vi "Stream to TDMS Files.vi"() -> ()   [LabVIEW 2023]
doc: "The Stream to TDMS File example shows how to save images to a TDMS file when using a grab acquisition. The TDMS API has been optimized to take advantage of asynchronous writes, parallel background workers, disk reservation, and disable buffering to improve write perfromance. Read the comments on the block diagram of this VI to learn more about these optimization options."
uses:
  SubVIs/Grab Manager Mode.ctl
  SubVIs/TDMS Write Settings.ctl
  <vilib>/vision/Image Controls.llb/IMAQ Image.ctl
  <vilib>/vision/driver/IMAQdx.llb/IMAQdx Buffer Number Mode.ctl
  <vilib>/Utility/High Resolution Relative Seconds.vi
  SubVIs/TDMS File Initialization (Write).vi
  <vilib>/vision/EDVR.llb/IMAQ ImageToEDVR.vi
  <vilib>/vision/EDVR.llb/IMAQ ImageToEDVR 1D U8.vi
  <vilib>/vision/EDVR.llb/IMAQ ImageToEDVR 1D I16.vi
  <vilib>/vision/EDVR.llb/IMAQ ImageToEDVR 1D U32.vi
  <vilib>/vision/EDVR.llb/IMAQ ImageToEDVR 1D U16.vi
  <vilib>/vision/driver/NI_Vision_Acquisition_Software.lvlib
  <resource>/objmgr/imaqdx.rc
panel:
  out "Optimizations":T1
  in  "Skip Count":u32
  out "Images Saved Per Second":dbl
  out "Images Acquired Per Second":dbl
  in  "Images per TDMS":i64=10000
  out "Write Speed":dbl(graph) caption="Image File Write Speed"
  out "Destination Folder":path
  out "Images Behind":u32
  in  "Number of Images":i32=30
  in  "Camera Name":refnum<k21> caption="IMAQdx Session"
  in  "Stop":bool
  # "Overview: Demonstrates how to stream images to TDMS files when using a grab acquisition.\nRequirements: Vision Acquisition Software\nInstructions:\n1. Select the Camera Name\n2. Run the VI\n3. Increase the Skip Count if Images Behind is greater than 0."
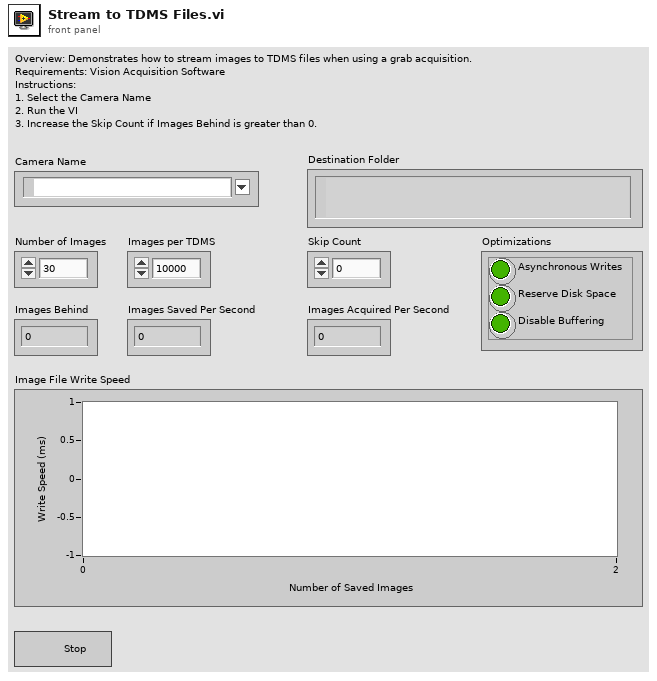
[diagram p1: front panel]
types:
  T1 = cluster{"Asynchronous Writes":bool, "Reserve Disk Space":bool, "Disable Buffering":bool}
  T2 = typedef "TDMS Write Settings.ctl" = cluster{"Asynchronous":bool, "Disable Buffering if Supported":bool, "Reserved Images":i64, "Fail if Reservation Fails":bool}
  T3 = typedef "Grab Manager Mode.ctl" = enum16{"Create Processing Images", "Lock", "Add Acquired Image", "Get Acquired Image", "Unlock", "Dispose Processing Images"}
  T4 = cluster{"Number of Processing Images":u32, "Image Border Size":u32}
  T5 = typedef "IMAQdx.ctl" = refnum<k21>
  T6 = typedef "IMAQ Image.ctl" = refnum<image>
  T7 = typedef "Image Type" = u32
  T8 = cluster{"Image Type":T7, "Async File Format":bool}
  T9 = cluster{"Asynchronous Write":bool, "Reserve Disk Space":bool, "Disable Buffering":bool}
  T10 = typedef "NI_Vision_Acquisition_Software.lvlib/IMAQdx Buffer Number Mode.ctl" = enum32{"Next", "Last", "Buffer Number", "Every", "Last New"}
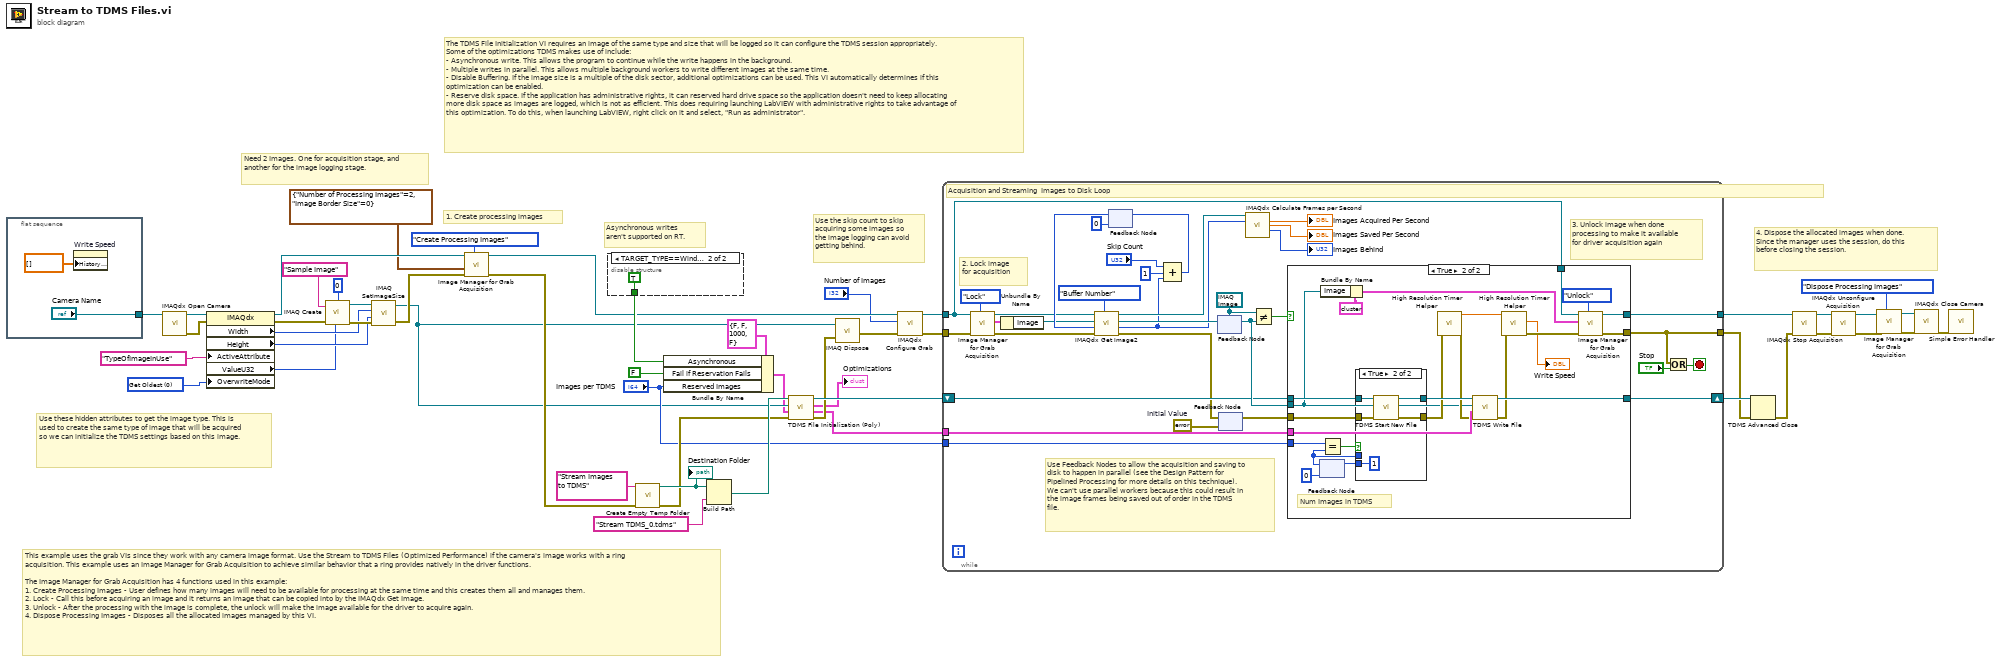
[diagram p0: block diagram]
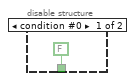
[diagram p2: hidden frame]
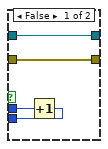
[diagram p4: hidden frame]
diagram:
  w4 = u32 0 items=["Get Oldest"=0, "Fail"=2, "Get Newest"=3] ("OverwriteMode")
  # "4. Dispose the allocated images when done. Since the manager uses the session, do this before closing the session."
  # "1. Create processing images"
  # "This example uses the grab VIs since they work with any camera image format. Use the Stream to TDMS Files (Optimized Performance) if the camera's image works with a ring acquisition. This example uses an Image Manager for Grab Acquisition to achieve similar behavior that a ring provides natively in the driver functions.\n\nThe Image Manager for Grab Acquisition has 4 functions used in this example:\n1. Create Processing Images - User defines how many images will need to be available for processing at the same time and this creates them all and manages them.\n2. Lock - Call this before acquiring an image and it returns an image that can be copied into by the IMAQdx Get Image.\n3. Unlock - After the processing with the image is complete, the unlock will make the image available for the driver to acquire again.\n4. Dispose Processing Images - Disposes all the allocated images managed by this VI."
  # "Need 2 Images. One for acquisition stage, and another for the image logging stage."
  # "The TDMS File Initialization VI requires an image of the same type and size that will be logged so it can configure the TDMS session appropriately. Some of the optimizations TDMS makes use of include:\n- Asynchronous write. This allows the program to continue while the write happens in the background.\n- Multiple writes in parallel. This allows multiple background workers to write different images at the same time.\n- Disable Buffering. If the image size is a multiple of the disk sector, additional optimizations can be used. This VI automatically determines if this optimization can be enabled.\n- Reserve disk space. If the application has administrative rights, it can reserved hard drive space so the application doesn't need to keep allocating more disk space as images are logged, which is not as efficient. This does requiring launching LabVIEW with administrative rights to take advantage of this optimization. To do this, when launching LabVIEW, right click on it and select, \"Run as administrator\"."
  # "Asynchronous writes aren't supported on RT."
  # "Use the skip count to skip acquiring some images so the image logging can avoid getting behind."
  # "Use these hidden attributes to get the image type. This is used to create the same type of image that will be acquired so we can initialize the TDMS settings based on this image."
  n1 = flat-sequence {
    tunnel: ["Camera Name"] -> w50
    frame #0 {
      n2 = property on="Write Speed" class="WFChart (strict)"("History Data"=dbl[] []) -> ()  [unwired: 2 in, 2 out]
    }
  }
  n3 = call <vilib>:"IMAQdx Open Camera.vi"("Session In"=w50) -> ("error out"=w48:errorcluster, "Session Out"=w49:T5)  [unwired: 2 in, 7 out]
  n4 = property class="IMAQdx"(reference=w49, error in=w48, "ActiveAttribute"="TypeOfImageInUse", "OverwriteMode"=w4) -> (reference out=w20:T5, error out=w46:errorcluster, "Width"=w42:u32, "Height"=w41:u32, "ValueU32"=w40:u32)
  n5 = call "IMAQ Create"("Border Size"=0, "Image Name"="Sample Image", "Image Type"=w40, "error in (no error)"=w46) -> ("New Image"=w43:T6, "error out"=w44:errorcluster)  [unwired: 1 out]
  n6 = call "IMAQ SetImageSize"("error in (no error)"=w44, "Y Resolution"=w41, "X Resolution"=w42, "Image"=w43) -> ("error out"=w19:errorcluster, "Image Out"=w6:T6)  [unwired: 1 in]
  n7 = call "Image Manager for Grab Acquisition.vi"("Mode"=Grab_Manager_Mode."Create Processing Images", "error in (no error)"=w19, "Init Settings"=T4 {"Number of Processing Images"=2, "Image Border Size"=0}, "Session In"=w20) -> ("error out"=w18:errorcluster, "Session Out"=w16:T5)  [unwired: 4 in, 2 out]
  n8 = disable-structure shown="TARGET_TYPE==Windows" {
    disable-tunnel: [FALSE ("Asynchronous") TRUE ("Asynchronous")] -> w22
    frame condition #0 {
    }
    frame condition #1 (active) {
    }
  }
  n9 = call "Create Empty Temp Folder.vi"("error in (no error)"=w18, "Folder Name"="Stream Images to TDMS") -> ("error out"=w30:errorcluster, "Empty Temp Folder"=w35:path)  [unwired: 8 in]
  "Destination Folder" <- w35
  n10 = Bundle By Name(cluster=T2 {"Asynchronous"=FALSE, "Disable Buffering if Supported"=FALSE, "Reserved Images"=1000, "Fail if Reservation Fails"=FALSE} ("Write Settings"), "Asynchronous"=w22, "Fail if Reservation Fails"=FALSE, "Reserved Images"="Images per TDMS") -> (w5:T2)
  n11 = Build Path(base path=w35, name or relative path="Stream TDMS_0.tdms") -> (appended path=w32:path)
  n12 = call-poly "TDMS File Initialization (Poly).vi"("error in (no error)"=w30, "Write Settings"=w5, "Image In"=w6, "File Path"=w32) -> ("error out"=w29:errorcluster, "Write Settings Out"=w27:T8, "Optimizations Configured"=→"Optimizations":T9, "TDMS Refnum Out"=w33:refnum<k34>)  [unwired: 4 in]
  n13 = call "IMAQ Dispose"("Image"=w6, "error in (no error)"=w29) -> ("error out"=w15:errorcluster)  [unwired: 4 in]
  n14 = call <vilib>:"IMAQdx Configure Grab.vi"("error in"=w15, "Number of Buffers"="Number of Images", "Session In"=w16) -> ("error out"=w12:errorcluster, "Session Out"=w13:T5)  [unwired: 7 in]
  n15 = while {
    tunnel: w12 -> [w60]
    tunnel: w13 -> [w61]
    tunnel: [w85] -> w37
    tunnel: [w78] -> w25
    shift-right: [w86] -> w26
    shift-left: w33 -> [w76]
    tunnel: "Images per TDMS" -> [w75]
    tunnel: w27 -> [w77]
    stop <- w80 stop-if-true
    w55 = errorcluster {"status"=FALSE, "code"=0, "source"=""}  # Initial Value
    w83 = T6 refnum ("Image Out")
    # "3. Unlock image when done processing to make it available for driver acquisition again"
    # "2. Lock image for acquisition"
    # "Use Feedback Nodes to allow the acquisition and saving to disk to happen in parallel (see the Design Pattern for Pipelined Processing for more details on this technique). We can't use parallel workers because this could result in the image frames being saved out of order in the TDMS file."
    # "Acquisition and Streaming  Images to Disk Loop"
    n16 = call "Image Manager for Grab Acquisition.vi"("Mode"=Grab_Manager_Mode."Lock", "error in (no error)"=w60, "Session In"=w61) -> ("error out"=w59:errorcluster, "Image Settings Out"=w57:cluster{"Image":T6, "Buffer Number":u32}, "Session Out"=w58:T5)  [unwired: 5 in, 1 out]
    n17 = Unbundle By Name(w57) -> ("Image"=w56:T6)
    n18 = feedback #1(u32 0) -> (w68:u32)
    n19 = call <vilib>:"IMAQdx Get Image2.vi"("Buffer Number Mode (Next)"=IMAQdx_Buffer_Number_Mode."Buffer Number" ("Buffer Number Mode"), "error in"=w59, "Buffer Number In"=w68, "Image In"=w56, "Session In"=w58) -> ("error out"=w63:errorcluster, "Buffer Number Out"=w64:u32, "Image Out"=w65:T6, "Session Out"=w66:T5)  [unwired: 3 in]
    n20 = Compound Arithmetic op=ADD("Skip Count", u32 1 ("value"), w64) -> (w71:u32)
    n21 = feedback-in #1(w71) -> ()
    n22 = feedback-in #2(w65) -> ()
    n23 = feedback #2(w83) -> (w81:T6)
    n24 = feedback-in #3(w63) -> ()
    n25 = feedback #3(w55) -> (w84:errorcluster)
    n26 = call <vilib>:"IMAQdx Calculate Frames per Second.vi"("Session In"=w66, "Buffer Number"=w64) -> ("Acquired Frames per Second"=→"Images Acquired Per Second":dbl, "Processed Frames per Second"=→"Images Saved Per Second":dbl, "Images Behind"=→"Images Behind":i32)  [unwired: 7 in, 4 out]
    n27 = Not Equal?(x=w83, y=w81) -> (x != y?=w82:bool)
    n28 = case shown="True" w82 {
      tunnel: w76 -> [w88 w110]
      tunnel: w81 -> [_ w93]
      tunnel: w84 -> [w89 w108]
      tunnel: [w88 w113] -> w86
      tunnel: [w90 w98] -> w85
      tunnel: w61 -> [w90 w95]
      tunnel: [w89 w97] -> w78
      tunnel: w77 -> [_ w112]
      tunnel: w75 -> [_ w106]
      frame False {
        # "First iteration doesn't have valid image for this pipelined stage."
      }
      frame True {
        # "Num Images in TDMS"
        n29 = feedback #4(i64 0) -> (w105:i64)
        n30 = Bundle By Name(cluster=cluster{"Image":T6, "Buffer Number":u32} {"Image"=refnum, "Buffer Number"=0} ("Image Settings In"), "Image"=w93) -> (w92:cluster{"Image":T6, "Buffer Number":u32})
        n31 = Equal?(x=w106, y=w105) -> (x = y?=w107:bool)
        n32 = case shown="True" w107 {
          tunnel: [w117 i64 1] -> w104
          tunnel: w110 -> [w116 w121]
          tunnel: [w116 w120] -> w109
          tunnel: w108 -> [w115 w118]
          tunnel: [w115 w119] -> w103
          tunnel: w105 -> [w114 _]
          frame False {
            n33 = Increment(x=w114) -> (x+1=w117:i64)
          }
          frame True {
            n34 = call "TDMS Start New File.vi"("error in"=w118, "Previous TDMS Refnum In"=w121) -> ("error out"=w119:errorcluster, "New TDMS Refnum Out"=w120:refnum<k34>)  [unwired: 8 in]
          }
        }
        n35 = feedback-in #4(w104) -> ()
        n36 = call "High Resolution Timer Helper.vi"("error in (no error)"=w103) -> ("error out"=w102:errorcluster, "Current Time"=w100:dbl)  [unwired: 8 in, 1 out]
        n37 = call "TDMS Write File.vi"("error in"=w102, "Write Settings"=w112, "Image"=w93, "TDMS Ref In"=w109) -> ("error out"=w101:errorcluster, "TDMS Ref Out"=w113:refnum<k34>)  [unwired: 6 in]
        n38 = call "High Resolution Timer Helper.vi"("error in (no error)"=w101, "Previous Time"=w100) -> ("error out"=w96:errorcluster, "Time Difference (ms)"=→"Write Speed":dbl)  [unwired: 7 in, 1 out]
        n39 = call "Image Manager for Grab Acquisition.vi"("Mode"=Grab_Manager_Mode."Unlock", "error in (no error)"=w96, "Image Settings In"=w92, "Session In"=w95) -> ("error out"=w97:errorcluster, "Session Out"=w98:T5)  [unwired: 4 in, 2 out]
      }
    }
    n40 = Or(x=w78, y="Stop") -> (x .or. y?=w80:bool)
  }
  n41 = TDMS Advanced Close(8:w25, 11:w26) -> (0:w24:errorcluster)  [unwired: 2 in, 1 out]
  n42 = call <vilib>:"IMAQdx Stop Acquisition.vi"("error in"=w24, "Session In"=w37) -> ("error out"=w38:errorcluster, "Session Out"=w39:T5)  [unwired: 8 out]
  n43 = call <vilib>:"IMAQdx Unconfigure Acquisition.vi"("error in"=w38, "Session In"=w39) -> ("error out"=w11:errorcluster, "Session Out"=w10:T5)  [unwired: 8 out]
  n44 = call "Image Manager for Grab Acquisition.vi"("Mode"=Grab_Manager_Mode."Dispose Processing Images", "error in (no error)"=w11, "Session In"=w10) -> ("error out"=w7:errorcluster, "Session Out"=w8:T5)  [unwired: 5 in, 2 out]
  n45 = call <vilib>:"IMAQdx Close Camera.vi"("error in"=w7, "Session In"=w8) -> ("error out"=w1:errorcluster)  [unwired: 9 out]
  n46 = call <vilib>:"Simple Error Handler.vi"("error in (no error)"=w1) -> ()  [unwired: 4 in, 5 out]
